vi "Write Detected_Current_ref.vi"(8 "error in (no error)":errorcluster, 10 "Detected_Current_ref":refnum<vi>, 11 "DIG_IO in":refnum<class "DIG_IO.lvclass">) -> (0 "error out":errorcluster, 3 "DIG_IO out":refnum<class "DIG_IO.lvclass">)   [LabVIEW 2019, in "DIG_IO.lvlib" / "DIG_IO.lvclass"]
uses:
  Library/DIG_IO.lvclass
  Library/DIG_IO.lvclass/DIG_IO.ctl
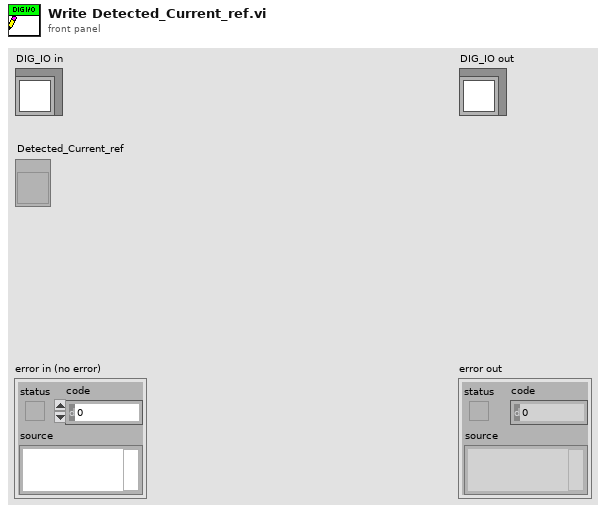
[diagram p1: front panel]
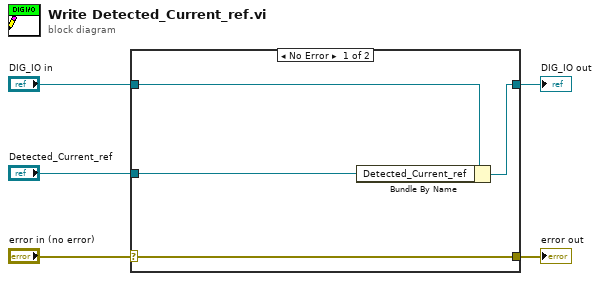
[diagram p0: block diagram]
diagram:
  n1 = case shown="No Error" "error in (no error)" {
    selector: "error in (no error)" -> [w9 w10]
    tunnel: [w9 w10] -> w4
    tunnel: [w7 w11] -> w2
    tunnel: "DIG_IO in" -> [w8 w11]
    tunnel: "Detected_Current_ref" -> [w6 _]
    frame No Error {
      n2 = Bundle By Name(cluster=w8, "Detected_Current_ref"=w6) -> (w7:refnum<class "DIG_IO.lvclass">)
    }
    frame Error {
    }
  }
  "error out" <- w4
  "DIG_IO out" <- w2
